vi "niRFSG Configure Output Enabled.vi"(0 "instrument handle":refnum<k15>, 7 "output enabled":bool, 11 "error in":errorcluster {"code" format="%.0x"}) -> (4 "instrument handle out":refnum<k15>, 15 "error out":errorcluster {"code" format="%.0x"})   [LabVIEW 2014]
doc: "Enables or disables signal output. Setting <B>output enabled</B> to FALSE while in the Generation state attenuates the generated signal so that no signal is output.\n\n<B>Supported Devices</B>: NI 5610, NI 5644R/5645R/5646R, NI 5650/5651/5652/5654/5654 with NI 5696, NI 5670/5671/5672/5673/5673E, NI 5840"
uses:
  niRFSG.dll
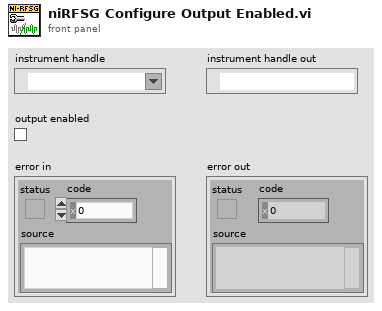
[diagram p1: front panel]
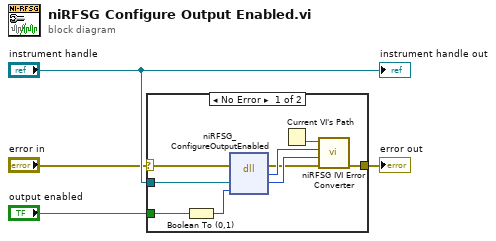
[diagram p0: block diagram]
diagram:
  n1 = case shown="No Error" "error in" {
    selector: "error in" -> [w6 w14]
    tunnel: "instrument handle" -> [w13 _]
    tunnel: [w12 w14] -> w3
    tunnel: "output enabled" -> [w5 _]
    frame No Error {
      n2 = Boolean To (0,1)(Boolean=w5) -> (0, 1=w11:i16)
      n3 = dll-call lib="niRFSG**.*" fn="niRFSG_ConfigureOutputEnabled"(error in=w6, "instrument handle"=w13, "Output Enabled"=w11) -> (error out=w7:errorcluster, "status"=w10:i32, "instrument handle"=w8:u32)  [unwired: 3 in, 1 out]
      n4 = Current VI's Path() -> (path=w9:path)
      n5 = call "niRFSG IVI Error Converter.vi"("error in"=w7, "instrument handle"=w8, "IVI error code"=w10, "path to VI"=w9) -> ("error out"=w12:errorcluster)  [unwired: 7 in]
    }
    frame Error {
    }
  }
  "error out" <- w3
  "instrument handle out" <- "instrument handle"
